vi "Encoder (SubVI).vi"(8 "error in (no error)":errorcluster, 11 "Reset?":bool) -> (0 "error out":errorcluster)   [LabVIEW 2017]
uses:
  <vilib>/myRIO/Instrument Drivers/Onboard IO/Encoder/vis/Read.vi
  <vilib>/myRIO/Instrument Drivers/Onboard IO/Encoder/vis/Smart Open.vi
  <vilib>/Utility/error.llb/Error Cluster From Error Code.vi
  <vilib>/myRIO/Common/Instrument Driver Framework/myRIO v1.0/Encoder/vis/myRIO v1.0 Read Encoder.vi
  Projects/Auto control/Inputs.vi
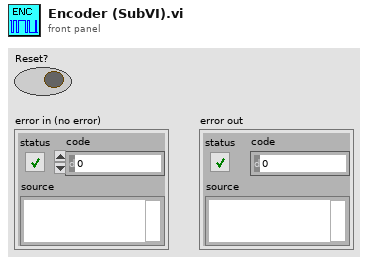
[diagram p1: front panel]
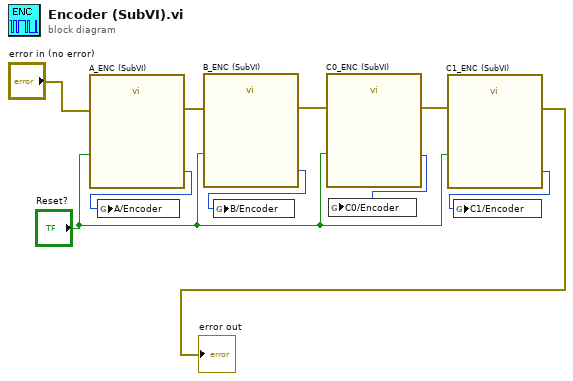
[diagram p0: block diagram]
diagram:
  n1 = call "A_ENC (SubVI).vi"("Reset Counter"="Reset?", "error in (no error)"="error in (no error)") -> ("Counter Value"=w9:i32, "error out"=w1:errorcluster)  [unwired: 22 in, 2 out]
  n2 = global write "Inputs.vi" "A/Encoder"(w9) -> ()
  n3 = call "B_ENC (SubVI).vi"("Reset Counter"="Reset?", "error in (no error)"=w1) -> ("Counter Value"=w8:i32, "error out"=w3:errorcluster)  [unwired: 22 in, 2 out]
  n4 = global write "Inputs.vi" "B/Encoder"(w8) -> ()
  n5 = call "C0_ENC (SubVI).vi"("Reset Counter"="Reset?", "error in (no error)"=w3) -> ("Counter Value"=w7:i32, "error out"=w4:errorcluster)  [unwired: 22 in, 2 out]
  n6 = global write "Inputs.vi" "C0/Encoder"(w7) -> ()
  n7 = call "C1_ENC (SubVI).vi"("Reset Counter"="Reset?", "error in (no error)"=w4) -> ("Counter Value"=w6:i32, "error out"=→"error out":errorcluster)  [unwired: 22 in, 2 out]
  n8 = global write "Inputs.vi" "C1/Encoder"(w6) -> ()
